vi "Configure.vi"(8 "error in (no error)":errorcluster, 11 "LCR-Measurement in":refnum<class "LCR-Meas.lvclass">) -> (0 "error out":errorcluster, 3 "LCR-Measurement out":refnum<class "LCR-Meas.lvclass">)   [LabVIEW 2020, in "LCR-Meas.lvclass"]
doc: "Configure the measurements paramaters to sweep.\nThis should be a pop up interface invoked by the configure test button on the main panel."
uses:
  LCR-Meas.lvclass
panel:
  in  "Cancel Button":bool
  in  "OK Button":bool
  in  "Bias Voltage (V)":string="0:3/0.1,\n3:-3/0.1,\n-3:0/0.1"
  in  "Enable Bias":bool
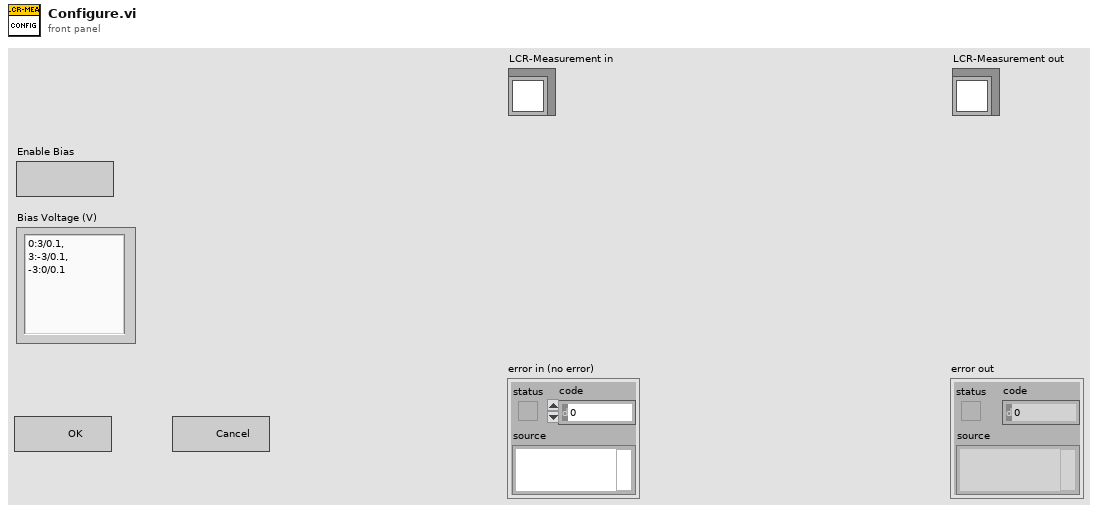
[diagram p1: front panel]
types:
  T1 = enum8{"Enabled", "Disabled", "Disabled and Grayed Out"}
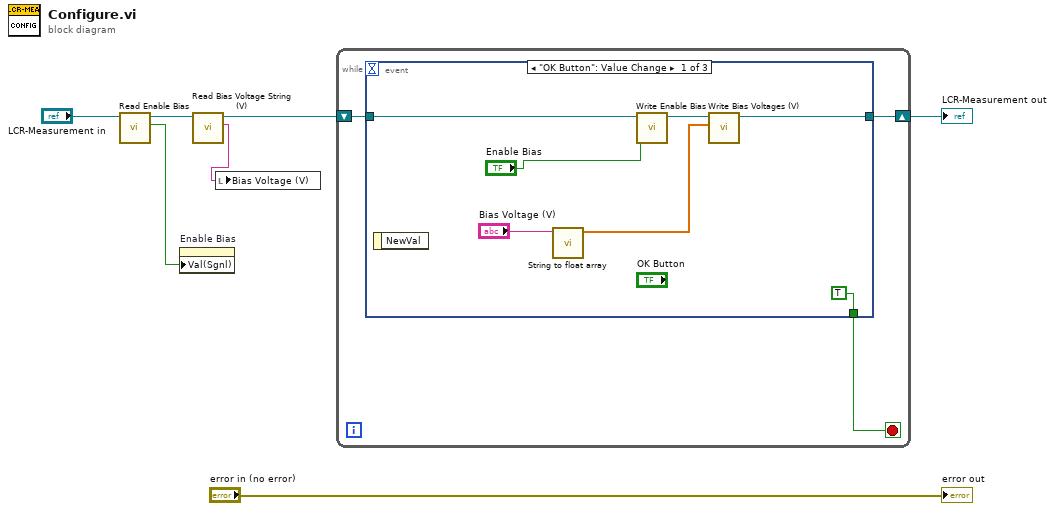
[diagram p0: block diagram]
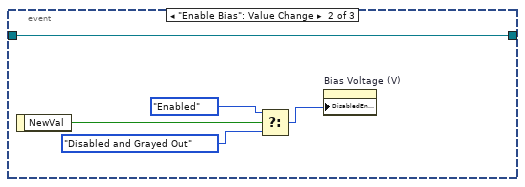
[diagram p2: hidden frame]
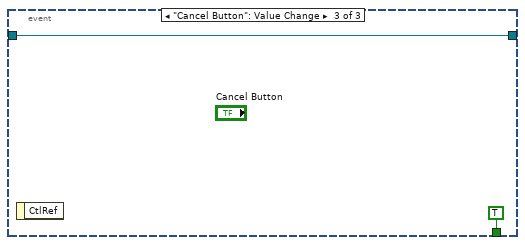
[diagram p3: hidden frame]
diagram:
  n1 = call-dynamic "Read Enable Bias.vi"("LCR-Measurement in"="LCR-Measurement in") -> ("Enable Bias"=w2:bool, "LCR-Measurement out"=w5:refnum<class "LCR-Meas.lvclass">)  [unwired: 9 in]
  n2 = property on="Enable Bias" class="Bool (strict)"("Val(Sgnl)"=w2) -> ()  [unwired: 2 in, 2 out]
  n3 = call-dynamic "Read Bias Voltage String (V).vi"("LCR-Measurement in"=w5) -> ("Bias Voltage String (V)"=w1:string, "LCR-Measurement out"=w3:refnum<class "LCR-Meas.lvclass">)  [unwired: 9 in]
  n4 = local write "Bias Voltage (V)"(w1) -> ()
  n5 = while {
    shift-right: [w9] -> w6
    shift-left: w3 -> [w10]
    stop <- w8 stop-if-true
    n6 = event shown="[0] \"OK Button\": Value Change" {
      selector: _ -> [_ _ _]
      dyn-events: _ -> [_ _ _]
      timeout: _ -> [_ _ _]
      tunnel: w10 -> [w14 w22 w23]
      tunnel: [w12 w22 w23] -> w9
      tunnel: [TRUE _ TRUE] -> w8
      event "OK Button": Value Change {
        n7 = event-data() -> ()  [unwired: 1 in, 1 out]
        n8 = call "String to float array.vi"("String"="Bias Voltage (V)") -> ("Array - Numeric"=w13:dbl[])  [unwired: 9 in, 1 out]
        n9 = call-dynamic "Write Enable Bias.vi"("Enable Bias"="Enable Bias", "LCR-Measurement in"=w14) -> ("LCR-Measurement out"=w16:refnum<class "LCR-Meas.lvclass">)  [unwired: 9 in]
        n10 = call-dynamic "Write Bias Voltages (V).vi"("Bias Voltages (V)"=w13, "LCR-Measurement in"=w16) -> ("LCR-Measurement out"=w12:refnum<class "LCR-Meas.lvclass">)  [unwired: 9 in]
      }
      event "Enable Bias": Value Change {
        n11 = event-data() -> ("NewVal"=w20:bool)  [unwired: 1 in]
        n12 = Select(t=T1."Enabled" ("Disabled"), s=w20, f=T1."Disabled and Grayed Out" ("Disabled")) -> (s? t:f=w18:T1)
        n13 = property on="Bias Voltage (V)" class="Str"("DisabledEnum"=w18) -> ()  [unwired: 2 in, 2 out]
      }
      event "Cancel Button": Value Change {
        n14 = event-data() -> ()  [unwired: 1 in, 1 out]
      }
    }
  }
  "LCR-Measurement out" <- w6
  "error out" <- "error in (no error)"
